vi "GdsLanguage_SetAttributes.vi"(2 "Attributes":T1, 5 "error in (no error)":errorcluster) -> (19 "error out":errorcluster)   [LabVIEW 2014]
doc: "This VI overwrites the attributes associated with the AcTranslator object reference and unlocks it for write access. If error in is set, the object is unlocked but its data will not be modified.\n\nIn order to use this VI, you must first successfully lock the object's data using the AcTranslator GetAttributesToModify VI.\n\n[GOOP 2.0.13]"
uses:
  <resource>/Framework/Providers/Open_GDS/ClassProviders/Common/GdsLanguage/private/GdsLanguage_ObjectAttributes.ctl
  <resource>/Framework/Providers/Open_GDS/ClassProviders/Common/GdsLanguage/GdsLanguage_LanguageID.ctl
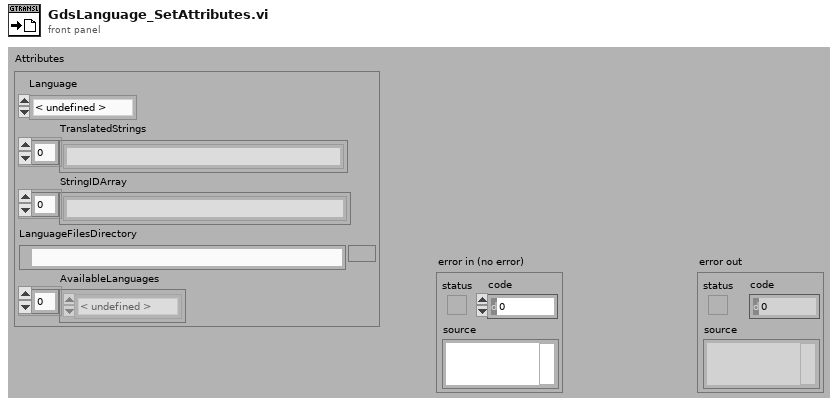
[diagram p1: front panel]
types:
  T1 = typedef "GdsLanguage_ObjectAttributes.ctl" = cluster{"Language":T2, "TranslatedStrings":string[], "StringIDArray":string[], "LanguageFilesDirectory":path, "AvailableLanguages":T2[]}
  T2 = typedef "GdsLanguage_LanguageID.ctl" = enum16{"< undefined >", "aa", "ab", "af", "am", "ar", "as", "ay", "az", "ba", "be", "bg", "bh", "bi", "bn", "bo", "br", "ca", "co", "cs", "cy", "da", "de", "dz", "el", "en", "eo", "es", "et", "eu", "fa", "fi", "fj", "fo", "fr", "fy", "ga", "gd", "gl", "gn", "gu", "gv", "ha", "he", "hi", "hr", "hu", "hy", "ia", "id", "ie", "ik", "is", "it", "iu", "ja", "jv", "ka", "kk", "kl", "km", "kn", "ko", "ks", "ku", "ky", "la", "li", "ln", "lo", "lt", "lv", "mg", "mi", "mk", "ml", "mn", "mo", "mr", "ms", "mt", "my", "na", "ne", "nl", "no", "oc", "om", "or", "pa", "pl", "ps", "pt", "qu", "rm", "rn", "ro", "ru", "rw", "sa", "sd", "sg", "sh", "si", "sk", "sl", "sm", "sn", "so", "sq", "sr", "ss", "st", "su", "sv", "sw", "ta", "te", "tg", "th", "ti", "tk", "tl", "tn", "to", "tr", "ts", "tt", "tw", "ug", "uk", "ur", "uz", "vi", "vo", "wo", "xh", "yi", "yo", "zh", "zu"}
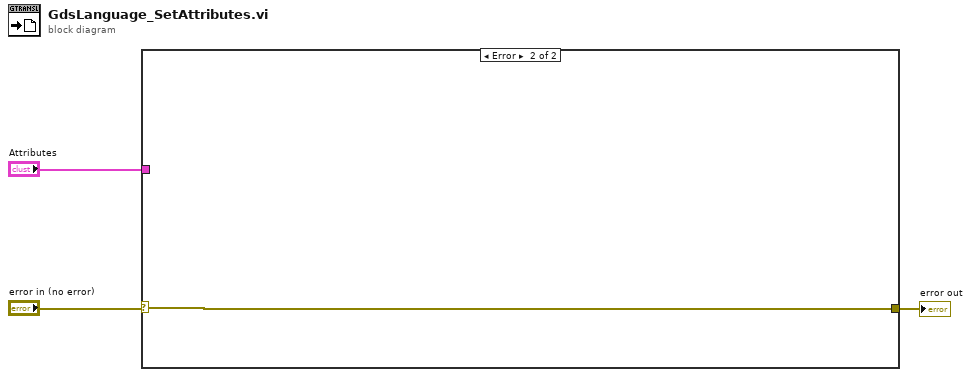
[diagram p0: block diagram]
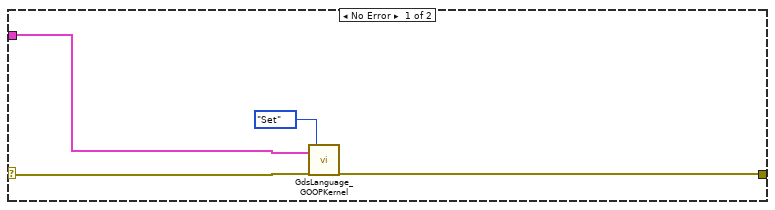
[diagram p2: hidden frame]
diagram:
  n1 = case shown="Error" "error in (no error)" {
    selector: "error in (no error)" -> [w7 w8]
    tunnel: "Attributes" -> [w6 _]
    tunnel: [w5 w8] -> w2
    frame No Error {
      n2 = call <resource>:"GdsLanguage_GOOPKernel.vi"("Data in"=w6, "error in (no error)"=w7, "Action"=enum16{"Get", "Set"}."Set") -> ("error out"=w5:errorcluster)  [unwired: 15 in, 1 out]
    }
    frame Error {
    }
  }
  "error out" <- w2
